vi "New Textbox.vi"(5 "Resize policy":T1, 6 "Size":T3={"W"=500.0, "H"=100.0}, 7 "Position":T4, 8 "error in (no error)":errorcluster, 9 "Text formatting":T2={"Font"="Arial", "Size"=18.0, "Italic"=FALSE, "Bold"=FALSE, "Underline"=FALSE, "Color"=0}, 10 "Text":string, 11 "Slide refnum":refnum<k7>) -> (0 "error out":errorcluster, 2 "Textbox refnum out":refnum<k7>, 3 "Slide refnum out":refnum<k7>)   [LabVIEW 2020, in "lvpptx.lvlib"]
uses:
  lvpptx.lvlib
  Position.ctl
  Size.ctl
  Font.ctl
  Textframe Resize Policy.ctl
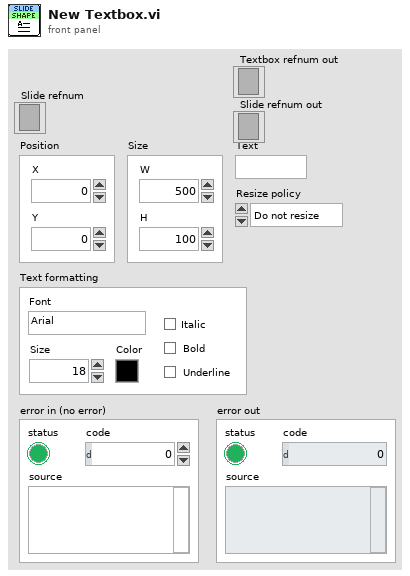
[diagram p1: front panel]
types:
  T1 = typedef "Textframe Resize Policy.ctl" = enum16{"Do not resize", "Expand horizontally", "Expand vertically"}
  T2 = typedef "lvpptx.lvlib/Font.ctl" = cluster{"Font":string, "Size":dbl, "Italic":bool, "Bold":bool, "Underline":bool, "Color":u32}
  T3 = typedef "lvpptx.lvlib/Size.ctl" = cluster{"W":dbl, "H":dbl}
  T4 = typedef "lvpptx.lvlib/Position.ctl" = cluster{"X":dbl, "Y":dbl}
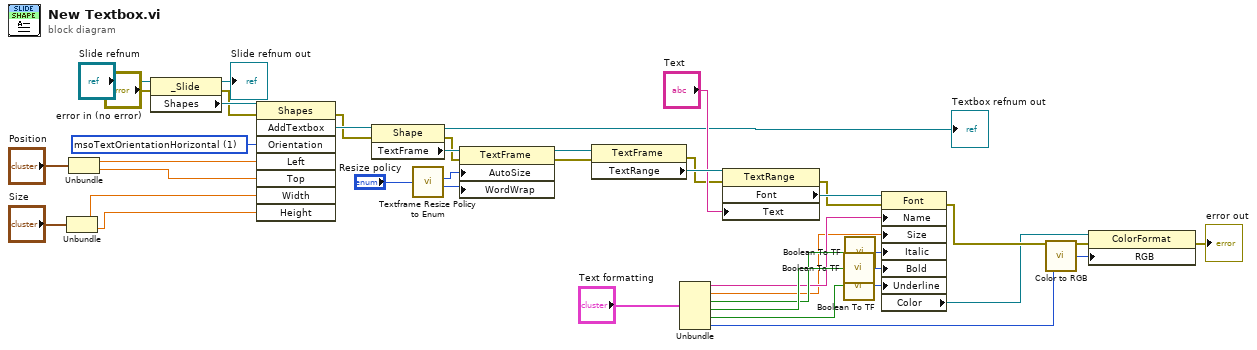
[diagram p0: block diagram]
diagram:
  w28 = 1 items=["msoTextOrientationMixed"=-2, "msoTextOrientationHorizontal"=1, "msoTextOrientationUpward"=2, "msoTextOrientationDownward"=3, "msoTextOrientationVerticalFarEast"=4, "msoTextOrientationVertical"=5, "msoTextOrientationHorizontalRotatedFarEast"=6] ("Orientation")
  n1 = Unbundle("Size") -> ("W"=w34:dbl, "H"=w35:dbl)
  n2 = Unbundle("Position") -> ("X"=w38:dbl, "Y"=w37:dbl)
  n3 = property class="_Slide"(reference="Slide refnum", error in="error in (no error)") -> (reference out=→"Slide refnum out":refnum<k7>, error out=w20:errorcluster, "Shapes"=w40:refnum<k7>)
  n4 = invoke class="Shapes" method="AddTextbox"(reference=w40, error in=w20, "Orientation"=w28, "Left"=w38, "Top"=w37, "Width"=w34, "Height"=w35) -> (error out=w21:errorcluster, "AddTextbox"=w33:refnum<k7>)  [unwired: 1 in, 6 out]
  n5 = property class="Shape"(reference=w33, error in=w21) -> (reference out=→"Textbox refnum out":refnum<k7>, error out=w15:errorcluster, "TextFrame"=w16:refnum<k7>)
  n6 = call "Textframe Resize Policy to Enum.vi"("Resize policy"="Resize policy") -> ("AutoSize"=w9:i32, "WordWrap"=w8:i32)  [unwired: 2 in]
  n7 = property class="TextFrame"(reference=w16, error in=w15, "AutoSize"=w9, "WordWrap"=w8) -> (reference out=w13:refnum<k7>, error out=w14:errorcluster)
  n8 = property class="TextFrame"(reference=w13, error in=w14) -> (error out=w22:errorcluster, "TextRange"=w32:refnum<k7>)  [unwired: 1 out]
  n9 = Unbundle("Text formatting") -> ("Font"=w6:string, "Size"=w5:dbl, "Italic"=w11:bool, "Bold"=w12:bool, "Underline"=w10:bool, "Color"=w18:u32)
  n10 = property class="TextRange"(reference=w32, error in=w22, "Text"="Text") -> (error out=w23:errorcluster, "Font"=w31:refnum<k7>)  [unwired: 1 out]
  n11 = call "Boolean To TF.vi"("Boolean"=w12) -> ("mso bool"=w3:i32)  [unwired: 4 in]
  n12 = call "Boolean To TF.vi"("Boolean"=w10) -> ("mso bool"=w2:i32)  [unwired: 4 in]
  n13 = call "Boolean To TF.vi"("Boolean"=w11) -> ("mso bool"=w4:i32)  [unwired: 4 in]
  n14 = property class="Font"(reference=w31, error in=w23, "Name"=w6, "Size"=w5, "Italic"=w4, "Bold"=w3, "Underline"=w2) -> (error out=w24:errorcluster, "Color"=w1:refnum<k7>)  [unwired: 1 out]
  n15 = call "Color to RGB.vi"("Color"=w18) -> ("32bit out"=w17:u32)  [unwired: 4 in]
  n16 = property class="ColorFormat"(reference=w1, error in=w24, "RGB"=w17) -> (error out=→"error out":errorcluster)  [unwired: 1 out]
